vi "Load ALL Waveforms.vi"(6 "Timeout (ms)":u32=15000, 8 "error in (no error)":errorcluster, 10 "Waveforms Operation (0: Save)":u16(ring) items=["Save", "Recall"], 11 "VISA resource name":refnum<visa-resource-name>="TCPIP0::A-N5182B-052670::inst0::INSTR") -> (0 "error out":errorcluster, 3 "VISA resource name out":refnum<visa-resource-name>="TCPIP0::A-N5182B-052670::inst0::INSTR")   [LabVIEW 2018]
doc: "(1) Stores from the internal BBG memory to the active media. (2) Loads all of the waveforms in the active media to the internal BBG memory. \nThe active media is either internal non-volatile memory storage media or an external storage media connected to the front-panel USB port.\n\n<b>Note:</b>\nThis VI is valid on N5172B that installs with <B>Option 653</B> or <B>Option 655</B>, or N5182B that installs with <B>Option 656</B> or <B>Option 657</B>, or N5162A, N5182A."
uses:
  Agilent PSG MXG Series/Agilent PSG MXG Series.lvlib
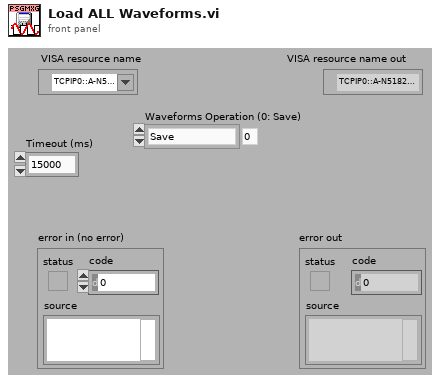
[diagram p1: front panel]
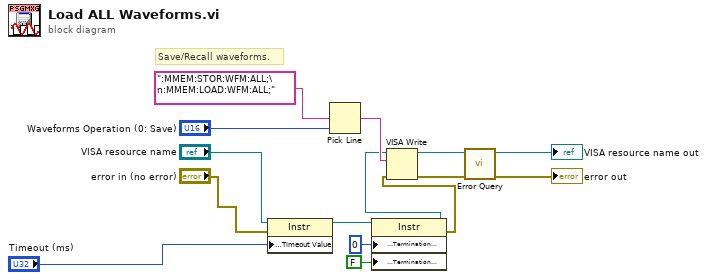
[diagram p0: block diagram]
diagram:
  # "Save/Recall waveforms."
  n1 = property class="Instr"(reference="VISA resource name", error in="error in (no error)", "General Settings:Timeout Value"="Timeout (ms)") -> (reference out=w7:refnum<visa-resource-name>)  [unwired: 1 out]
  n2 = Pick Line(multi-line string=":MMEM:STOR:WFM:ALL;\n:MMEM:LOAD:WFM:ALL;", line index="Waveforms Operation (0: Save)") -> (output string=w11:string)  [unwired: 1 in]
  n3 = property class="Instr"(reference=w7, "Message Based Settings:Termination Character"=u8 0, "Message Based Settings:Termination Character Enable"=FALSE) -> (reference out=w6:refnum<visa-resource-name>, error out=w2:errorcluster)  [unwired: 1 in]
  n4 = VISA Write(VISA resource name=w6, write buffer=w11, error in (no error)=w2) -> (VISA resource name out=w15:refnum<visa-resource-name>, error out=w14:errorcluster)  [unwired: 1 out]
  n5 = call "Error Query.vi"("error in (no error)"=w14, "VISA resource name"=w15) -> ("error out"=→"error out":errorcluster, "VISA resource name out"=→"VISA resource name out":refnum<visa-resource-name>)  [unwired: 8 out]
